vi "GetDisplayText.vi"(8 "Error In":errorcluster, 10 "Window":u8 min=1 max=2 step=1, 11 "Keithley 6482 In":refnum<visa-resource-name>) -> (0 "Error Out":errorcluster, 2 "Text (32 characters)":string, 3 "Keithley 6482 Out":refnum<visa-resource-name>)   [LabVIEW 2009, in "Keithley-6482-Visa.lvlib"]
uses:
  <instrlib>/Keithley-6482-Visa9.0/Keithley-6482-Visa.lvlib
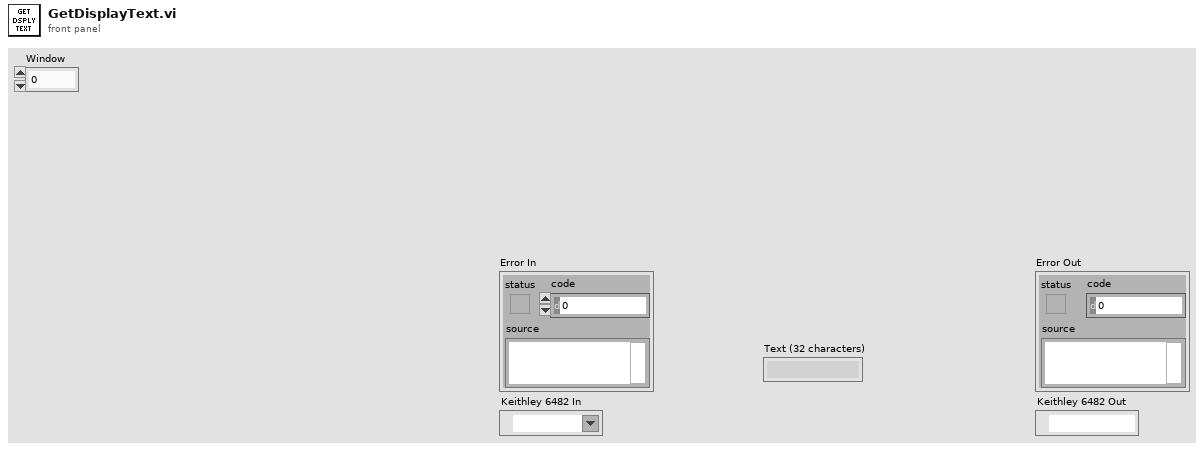
[diagram p1: front panel]
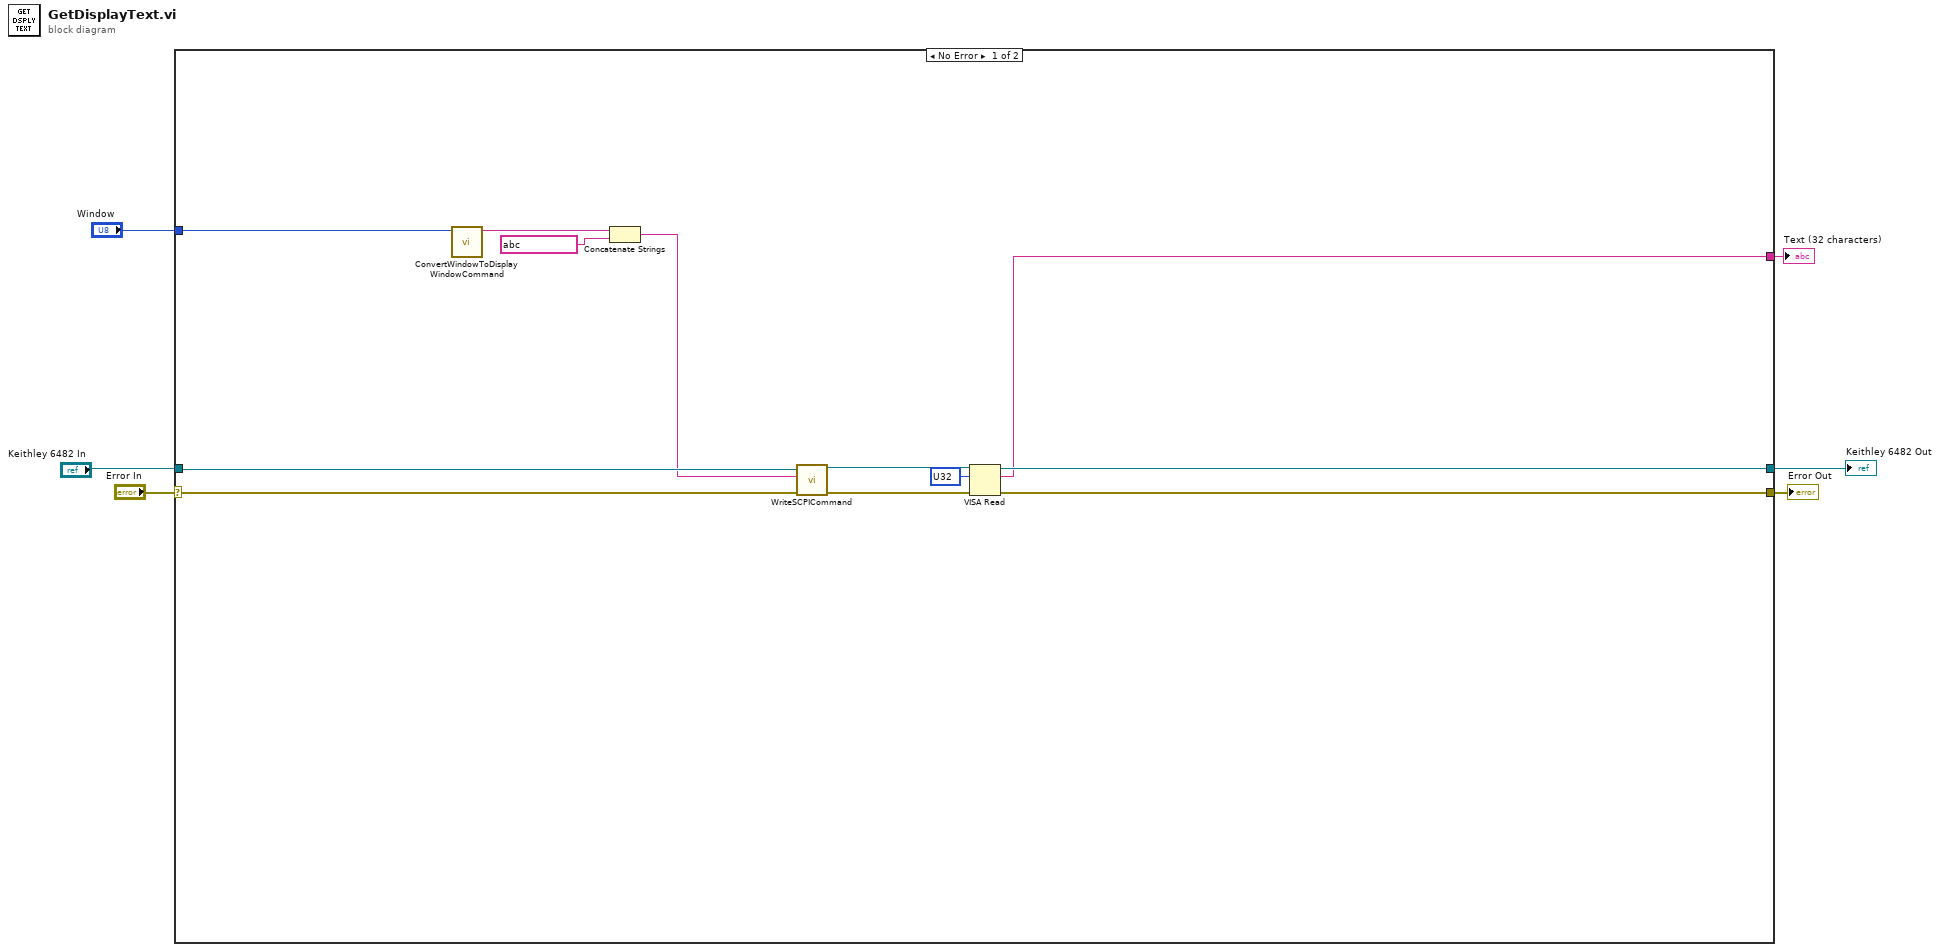
[diagram p0: block diagram]
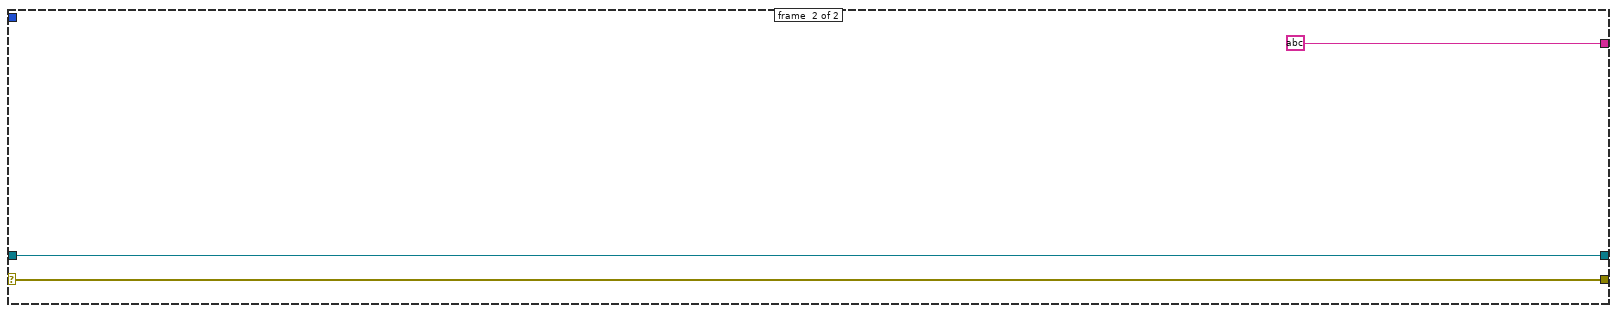
[diagram p2: hidden frame]
diagram:
  n1 = case shown="No Error" "Error In" {
    selector: "Error In" -> [w14 w20]
    tunnel: [w18 w20] -> w5
    tunnel: [w17 w21] -> w4
    tunnel: "Keithley 6482 In" -> [w15 w21]
    tunnel: [w11 string ?] -> w2
    tunnel: "Window" -> [w7 _]
    frame #0 {
      n2 = call <instrlib>:"ConvertWindowToDisplayWindowCommand.vi"("Window"=w7) -> ("Display Window Command"=w8:string)  [unwired: 10 in]
      n3 = Concatenate Strings(w8, string ?) -> (w9:string)
      n4 = call <instrlib>:"WriteSCPICommand.vi"("Error In"=w14, "SCPI Command"=w9, "Keithley 6482 In"=w15) -> ("Error Out"=w13:errorcluster, "Keithley 6482 Out"=w12:refnum<visa-resource-name>)  [unwired: 7 in]
      n5 = VISA Read(VISA resource name=w12, byte count=u32 ?, error in (no error)=w13) -> (VISA resource name out=w17:refnum<visa-resource-name>, read buffer=w11:string, error out=w18:errorcluster)  [unwired: 1 out]
    }
    frame #1 {
    }
  }
  "Error Out" <- w5
  "Keithley 6482 Out" <- w4
  "Text (32 characters)" <- w2
